vi "Event Structure.vi"() -> ()   [LabVIEW 2023]
doc: "The Event Structure example configures an event callback to handle every other acquired image. This allows the LabVIEW Event Structure to handle IMAQdx driver events in addition to user events."
uses:
  <vilib>/vision/driver/IMAQdx.llb/IMAQdx Acquisition Mode.ctl
  <vilib>/vision/driver/IMAQdx.llb/IMAQdx Buffer Number Mode.ctl
  <vilib>/vision/driver/NI_Vision_Acquisition_Software.lvlib
  <resource>/objmgr/imaqdx.rc
panel:
  out "Frame Rate":dbl
  out "Event Overrun":bool
  out "Image":T1(plugin-control)
  out "Buffer Number":u32
  in  "Camera Name":refnum<k21> caption="IMAQdx Session"
  in  "Stop":bool
  # "Overview: Demonstrates how to configure an event callback when an image is acquired that can be handled by a LabVIEW Event Structure.\nRequirements: Vision Acquisition Software\nInstructions: \n1. Select the Camera Name\n2. Run the VI"
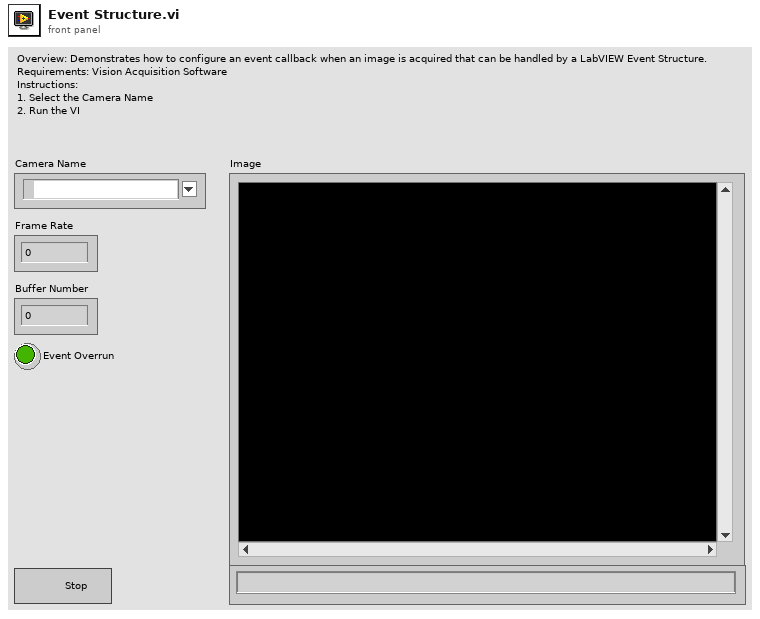
[diagram p1: front panel]
types:
  T1 = typedef "IMAQ Image.ctl" = refnum<image>
  T2 = typedef "NI_Vision_Acquisition_Software.lvlib/IMAQdx Acquisition Mode.ctl" = enum32{"One Shot", "Continuous"}
  T3 = typedef "IMAQdx.ctl" = refnum<k21>
  T4 = typedef "NI_Vision_Acquisition_Software.lvlib/IMAQdx Buffer Number Mode.ctl" = enum32{"Next", "Last", "Buffer Number", "Every", "Last New"}
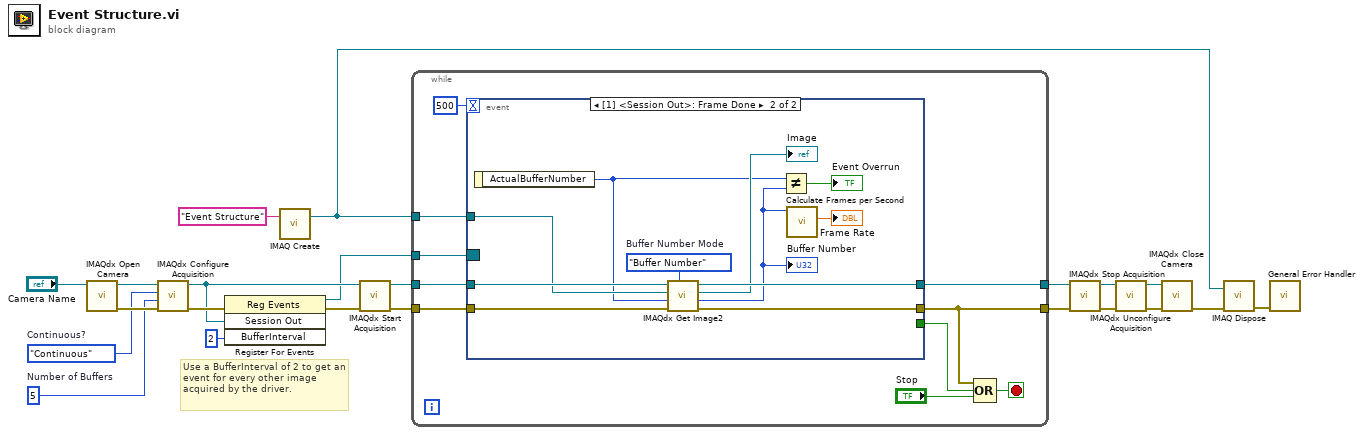
[diagram p0: block diagram]
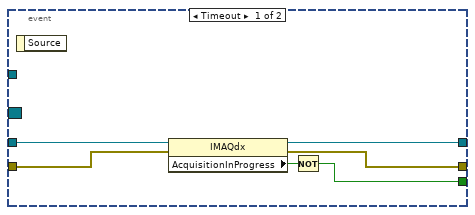
[diagram p2: hidden frame]
diagram:
  w17 = u32 5  # Number of Buffers
  w18 = IMAQdx_Acquisition_Mode."Continuous"  # Continuous?
  # "Use a BufferInterval of 2 to get an event for every other image acquired by the driver."
  n1 = call <vilib>:"IMAQdx Open Camera.vi"("Session In"="Camera Name") -> ("error out"=w20:errorcluster, "Session Out"=w22:T3)  [unwired: 2 in, 7 out]
  n2 = call <vilib>:"IMAQdx Configure Acquisition.vi"("error in"=w20, "Number of Buffers"=w17, "Continuous?"=w18, "Session In"=w22) -> ("error out"=w10:errorcluster, "Session Out"=w8:T3)  [unwired: 6 out]
  n3 = register-events(error in=w10, w8, u32 2 ("BufferInterval")) -> (reference out=w7:refnum<event-registration>, error out=w9:errorcluster)  [unwired: 1 in]
  n4 = call "IMAQ Create"("Image Name"="Event Structure") -> ("New Image"=w2:T1)  [unwired: 3 in, 2 out]
  n5 = call <vilib>:"IMAQdx Start Acquisition.vi"("error in"=w9, "Session In"=w8) -> ("error out"=w19:errorcluster, "Session Out"=w21:T3)  [unwired: 8 out]
  n6 = while {
    tunnel: [w28] -> w15
    tunnel: w19 -> [w30]
    tunnel: w21 -> [w31]
    tunnel: [w24] -> w16
    tunnel: w2 -> [w29]
    tunnel: w7 -> [w27]
    stop <- w32 stop-if-true
    n7 = event shown="[1] <Session Out>: Frame Done" {
      selector: w27 -> [_ _]
      dyn-events: _ -> [_ _]
      timeout: 500 -> [_ _]
      tunnel: w31 -> [w38 w49]
      tunnel: w30 -> [w37 w48]
      tunnel: w29 -> [_ w47]
      tunnel: [w36 w46] -> w28
      tunnel: [w35 w45] -> w24
      tunnel: [w33 _] -> w23
      event Timeout {
        n8 = event-data() -> ()  [unwired: 2 out]
        n9 = property class="IMAQdx"(reference=w38, error in=w37) -> (reference out=w36:T3, error out=w35:errorcluster, "AcquisitionInProgress"=w34:bool)
        n10 = Not(x=w34) -> (.not. x?=w33:bool)
      }
      event event #0x0 {
        w43 = IMAQdx_Buffer_Number_Mode."Buffer Number"  # Buffer Number Mode
        n11 = event-data() -> ("ActualBufferNumber"=w42:u32)  [unwired: 1 out]
        n12 = call <vilib>:"IMAQdx Get Image2.vi"("Buffer Number Mode (Next)"=w43, "error in"=w48, "Buffer Number In"=w42, "Image In"=w47, "Session In"=w49) -> ("error out"=w45:errorcluster, "Buffer Number Out"=w40:u32, "Image Out"=→"Image":T1, "Session Out"=w46:T3)  [unwired: 3 in]
        "Buffer Number" <- w40
        n13 = Not Equal?(x=w42, y=w40) -> (x != y?=→"Event Overrun":bool)
        n14 = call <vilib>:"Calculate Frames per Second.vi"("Buffer Number"=w40) -> ("Processed Frames/s"=→"Frame Rate":dbl)  [unwired: 8 in, 2 out]
      }
    }
    n15 = Compound Arithmetic op=OR(w24, w23, "Stop") -> (w32:bool)
  }
  n16 = call <vilib>:"IMAQdx Stop Acquisition.vi"("error in"=w16, "Session In"=w15) -> ("error out"=w11:errorcluster, "Session Out"=w12:T3)  [unwired: 8 out]
  n17 = call <vilib>:"IMAQdx Unconfigure Acquisition.vi"("error in"=w11, "Session In"=w12) -> ("error out"=w14:errorcluster, "Session Out"=w13:T3)  [unwired: 8 out]
  n18 = call <vilib>:"IMAQdx Close Camera.vi"("error in"=w14, "Session In"=w13) -> ("error out"=w4:errorcluster)  [unwired: 9 out]
  n19 = call "IMAQ Dispose"("Image"=w2, "error in (no error)"=w4) -> ("error out"=w3:errorcluster)  [unwired: 4 in]
  n20 = call <vilib>:"General Error Handler.vi"("error in (no error)"=w3) -> ()  [unwired: 2 in, 13 out]
